vi "Globals.vi"() -> ()   [LabVIEW 2015]
panel:
  out "THETA":dbl
  out "ezAFM Connected?":bool
  out "Status":string
  out "Scanning":bool
  out "Retracting":bool
  out "Approaching":bool
  out "Tip Approached?":bool
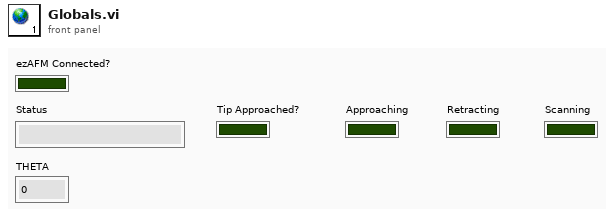
[diagram p1: front panel]
diagram:
